vi "LRange.vi"(0 "reference in":refnum<class "Redis.lvclass">, 1 "Key":string, 5 "Start Index":i32, 9 "Stop Index":i32, 11 "Error In":errorcluster) -> (4 "reference out":refnum<class "Redis.lvclass">, 8 "Elements":string[](array[string]), 15 "Error Out":errorcluster)   [LabVIEW 2020, in "Redis.lvclass"]
doc: "<b>LRANGE</b>\n\nReturns the specified elements of the list stored at key. The offsets start and stop are zero-based indexes, with 0 being the first element of the list (the head of the list), 1 being the next element and so on.\n\nThese offsets can also be negative numbers indicating offsets starting at the end of the list. For example, -1 is the last element of the list, -2 the penultimate, and so on."
uses:
  Redis.lvclass
  Redis.lvclass/Redis.ctl
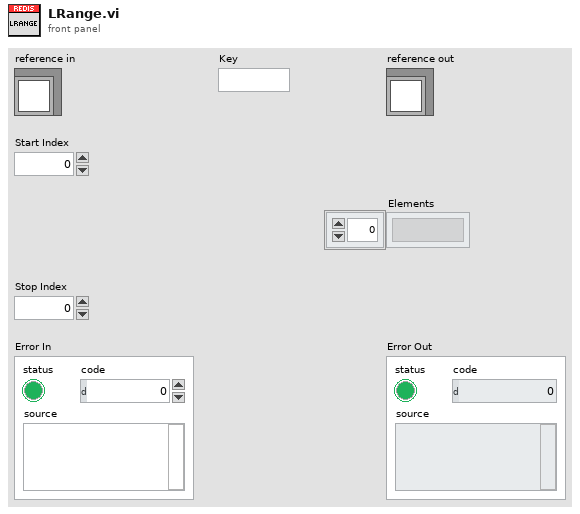
[diagram p1: front panel]
types:
  T1 = typedef "Redis.lvclass/RedisDataType.ctl" = cluster{"Reply Type":T2, "Integer":i64, "String":string, "Multibulk":variant[], "StringData":string[]}
  T2 = typedef "Redis.lvclass/ReplyDataTypeEnum.ctl" = enum16{"None", "Error", "Status", "Nil", "Integer", "String", "Multibulk"}
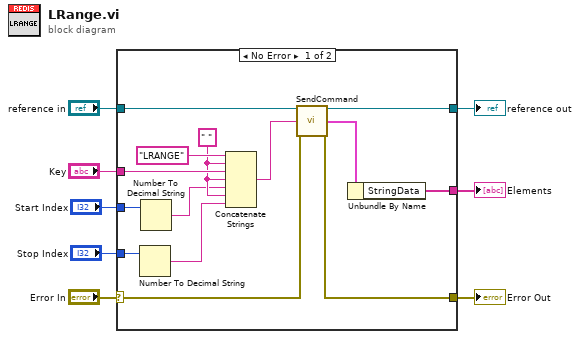
[diagram p0: block diagram]
diagram:
  n1 = case shown="No Error" "Error In" {
    selector: "Error In" -> [w20 w24]
    tunnel: [w10 w24] -> w7
    tunnel: [w22 w23] -> w5
    tunnel: "reference in" -> [w21 w23]
    tunnel: "Key" -> [w18 _]
    tunnel: "Start Index" -> [w15 _]
    tunnel: "Stop Index" -> [w14 _]
    tunnel: [w9 _] -> w1
    frame No Error {
      w13 = " "
      n2 = Number To Decimal String(number=w14) -> (decimal integer string=w11:string)  [unwired: 1 in]
      n3 = Number To Decimal String(number=w15) -> (decimal integer string=w12:string)  [unwired: 1 in]
      n4 = Concatenate Strings("LRANGE", w13, w18, w13, w12, w13, w11) -> (w17:string)
      n5 = call "SendCommand.vi"("reference in"=w21, "Command"=w17, "Error In"=w20) -> ("reference out"=w22:refnum<class "Redis.lvclass">, "Data"=w16:T1, "Error Out"=w10:errorcluster)  [unwired: 10 in]
      n6 = Unbundle By Name(w16) -> ("StringData"=w9:string[])
    }
    frame Error {
    }
  }
  "Error Out" <- w7
  "reference out" <- w5
  "Elements" <- w1
